vi "Perform Action.vi"(5 "Series Enqueuer":refnum<class "Message Enqueuer.lvclass">, 7 "Task Ident":string, 8 "error in":errorcluster, 9 "Input":variant, 10 "Point Ident":string, 11 "MSS in":refnum<class "MSS.lvclass">) -> (0 "error out":errorcluster, 1 "Output":variant, 2 "Task-Point Ident":string, 3 "MSS out":refnum<class "MSS.lvclass">)   [LabVIEW 2024, in "HAL.lvlib" / "MSS.lvclass"]
uses:
  MSS.lvclass
  MSS.lvclass/MSS.ctl
  <vilib>/ActorFramework/Message Enqueuer/Message Enqueuer.lvclass
  MAL/Series/ISeries Actor/ISeries Actor Messages/Perform Action on Target Msg/Perform Action on Target Msg.lvclass
  <vilib>/ActorFramework/Message Enqueuer/Message Priority.ctl
  MAL/Series/ISeries Actor/ISeries Actor Messages/Log Event Msg/Log Event Msg.lvclass
  Virtual Instruments/Virtual Instrument/Virtual Instrument.lvclass
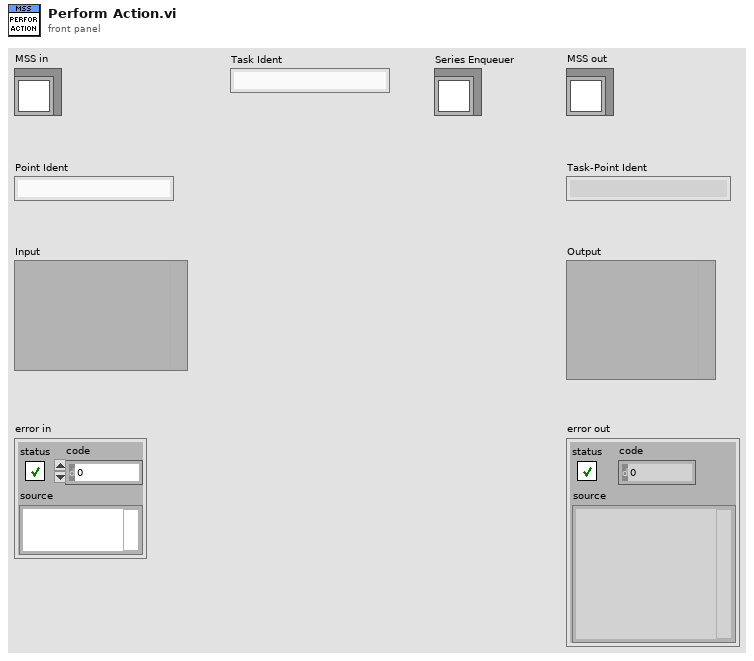
[diagram p1: front panel]
types:
  T1 = map{string, refnum<class "Virtual Instrument.lvclass">}
  T2 = typedef "Actor Framework.lvlib/Message Enqueuer.lvclass/Message Priority.ctl" = enum16{"Low", "Normal", "High"}
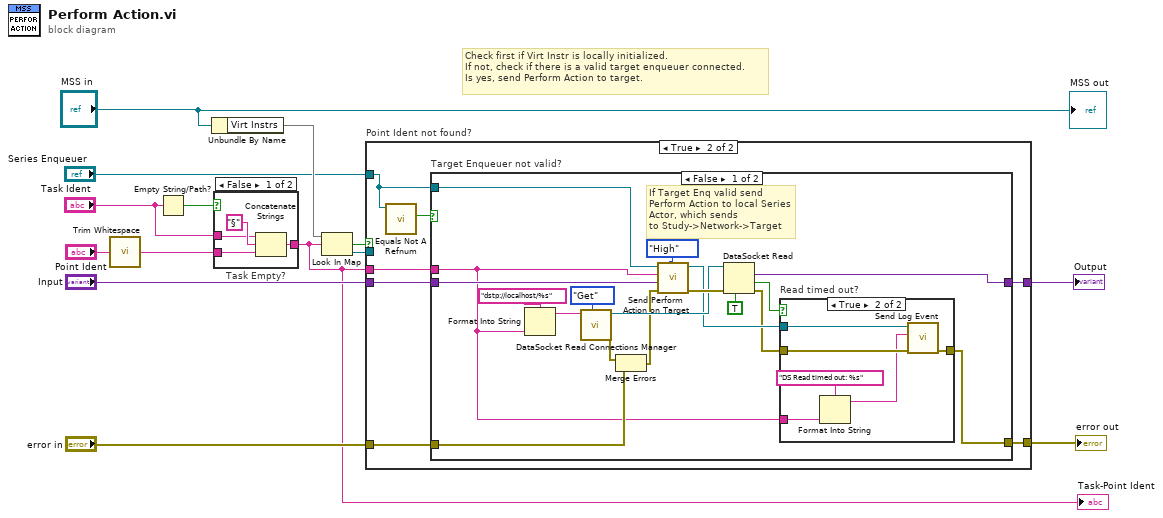
[diagram p0: block diagram]
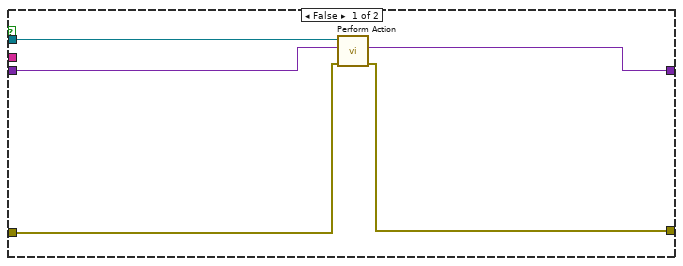
[diagram p3: hidden frame]
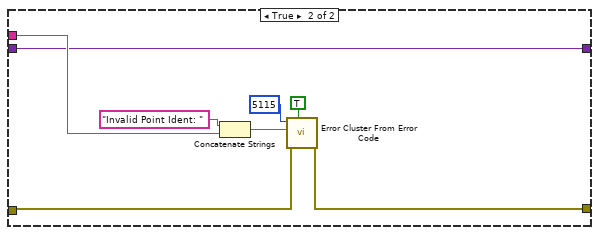
[diagram p5: hidden frame]
diagram:
  # "Check first if Virt Instr is locally initialized.\nIf not, check if there is a valid target enqueuer connected.\nIs yes, send Perform Action to target."
  n1 = call <vilib>:"Trim Whitespace.vi"("string"="Point Ident") -> ("trimmed string"=w2:string)  [unwired: 1 in]
  n2 = Empty String/Path?(string/path="Task Ident") -> (empty?=w5:bool)
  n3 = Unbundle By Name("MSS in") -> ("Virt Instrs"=w14:T1)
  n4 = case "Task Empty?" shown="False" w5 {
    tunnel: w2 -> [w15 w19]
    tunnel: [w18 w19] -> w1
    tunnel: "Task Ident" -> [w16 _]
    frame False {
      n5 = Concatenate Strings(w16, "§", w15) -> (w18:string)
    }
    frame True {
    }
  }
  "Task-Point Ident" <- w1
  n6 = Look In Map(map=w14, key=w1) -> (key not found?=w13:bool, value=w12:refnum<class "Virtual Instrument.lvclass">)  [unwired: 1 in]
  n7 = case "Point Ident not found?" shown="True" w13 {
    tunnel: "error in" -> [w21 w30]
    tunnel: w12 -> [w24 _]
    tunnel: [w20 w31] -> w8
    tunnel: [w23 w25] -> w9
    tunnel: "Input" -> [w22 w27]
    tunnel: "Series Enqueuer" -> [_ w28]
    tunnel: w1 -> [_ w26]
    frame False {
      n8 = call-dynamic "Perform Action.vi"("error in"=w21, "Input"=w22, "Virt Instr Base in"=w24) -> ("error out"=w20:errorcluster, "Output"=w23:variant)  [unwired: 6 in, 1 out]
    }
    frame True {
      n9 = call <vilib>:"Equals Not A Refnum.vi"("Message Enqueuer"=w28) -> ("Not a refnum?"=w29:bool)  [unwired: 10 in]
      n10 = case "Target Enqueuer not valid?" shown="False" w29 {
        tunnel: [w35 w61] -> w31
        tunnel: w30 -> [w49 w60]
        tunnel: w28 -> [w47 _]
        tunnel: w27 -> [w46 w58]
        tunnel: w26 -> [w34 w59]
        tunnel: [w39 w58] -> w25
        frame False {
          # "If Target Enq valid send Perform Action to local Series Actor, which sends\nto Study->Network->Target"
          n11 = Format Into String(format string="dstp://localhost/%s", w34) -> (resulting string=w42:string)  [unwired: 2 in, 1 out]
          n12 = call "DataSocket Read Connections Manager.vi"("Action"=enum16{"Get", "Close", "Close All"}."Get", "URL"=w42) -> ("error out"=w32:errorcluster, "connection id"=w40:refnum<k13>)  [unwired: 8 in]
          n13 = Merge Errors(w32, w49) -> (w33:errorcluster)
          n14 = call "Send Perform Action on Target.vi"("Message Priority (Normal)"=Message_Priority."High", "error in (no error)"=w33, "Input"=w46, "Task-Point Ident"=w34, "Message Enqueuer"=w47) -> ("error out"=w48:errorcluster, "Message Enqueuer out"=w37:refnum<class "Message Enqueuer.lvclass">)  [unwired: 5 in]
          n15 = DataSocket Read(6:TRUE ("wait for updated value (T)"), 8:w48, 11:w40) -> (0:w36:errorcluster, 1:w38:bool, 2:w39:variant)  [unwired: 2 in, 4 out]
          n16 = case "Read timed out?" shown="True" w38 {
            tunnel: w37 -> [_ w56]
            tunnel: w36 -> [w50 w55]
            tunnel: [w50 w54] -> w35
            tunnel: w34 -> [_ w53]
            frame False {
            }
            frame True {
              n17 = Format Into String(format string="DS Read timed out: %s", w53) -> (resulting string=w51:string)  [unwired: 2 in, 1 out]
              n18 = call "Send Log Event.vi"("error in (no error)"=w55, "Event Text"=w51, "Message Enqueuer"=w56) -> ("error out"=w54:errorcluster)  [unwired: 7 in, 1 out]
            }
          }
        }
        frame True {
          n19 = Concatenate Strings("Invalid Point Ident: " ("string"), w59) -> (w62:string)
          n20 = call <vilib>:"Error Cluster From Error Code.vi"("show call chain? (False)"=TRUE, "error in (no error)"=w60, "error message (\"\")"=w62, "error code (0)"=5115) -> ("error out"=w61:errorcluster)  [unwired: 5 in]
        }
      }
    }
  }
  "error out" <- w8
  "Output" <- w9
  "MSS out" <- "MSS in"
